vi "Message List FGV.vi"(6 "Action (Get)":enum16{"Get", "Add", "Reset"}(ring), 8 "error in (no error)":errorcluster, 11 "Message Object":refnum<class>) -> (0 "error out":errorcluster, 3 "Messages":string[](array[string]))   [LabVIEW 2017]
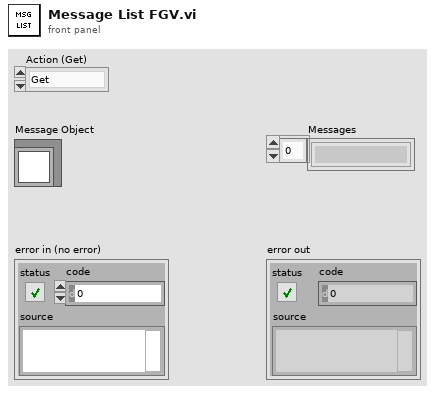
[diagram p1: front panel]
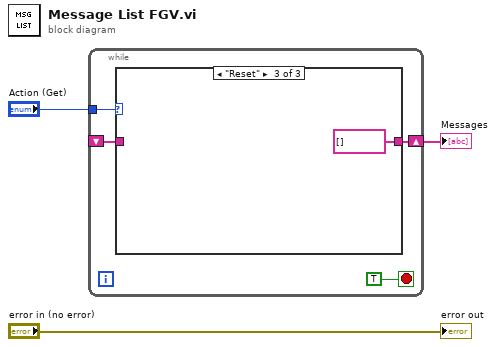
[diagram p0: block diagram]
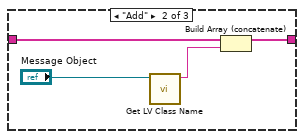
[diagram p3: hidden frame]
diagram:
  n1 = while {
    tunnel: "Action (Get)" -> [w6]
    shift-right: [w5] -> w1
    shift-left: _ -> [w4]
    stop <- TRUE stop-if-true
    n2 = case shown="\"Reset\"" w6 {
      tunnel: [w8 w11 string[] []] -> w5
      tunnel: w4 -> [w8 w12 _]
      frame "Get", Default {
      }
      frame "Add" {
        n3 = call <vilib>:"Get LV Class Name.vi"("object"="Message Object") -> ("class name"=w9:string)  [unwired: 9 in, 1 out]
        n4 = Build Array (concatenate)(w12, w9) -> (w11:string[])
      }
      frame "Reset" {
      }
    }
  }
  "Messages" <- w1
  "error out" <- "error in (no error)"
